vi "Работа с CVS( exel) файлом knob вариант 3.vi"() -> ()   [LabVIEW 2021]
uses:
  CSVtxtcluster.ctl
panel:
  out "record(s)":T1[](array[typedef]) {"Knob" scale=0.0..10.0}
  in  "datalog path (use dialog)":path
  in  "Cluster":T1 {"Knob" scale=0.0..10.0}
  in  "Knob":dbl(knob) scale=0.0..10.0
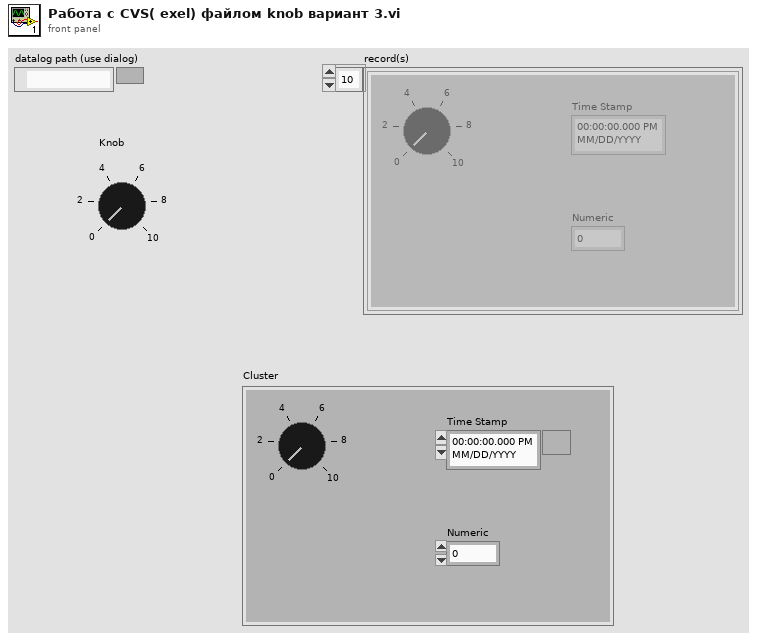
[diagram p1: front panel]
types:
  T1 = typedef "CSVtxtcluster.ctl" = cluster{"Knob":dbl, "Time Stamp":timestamp, "Numeric":dbl}
  T2 = enum16{"open", "replace", "create", "open or create", "replace or create", "replace or create with confirmation"}
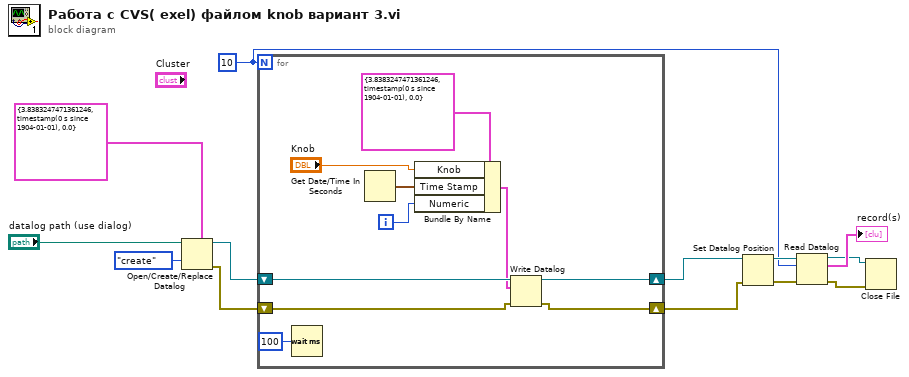
[diagram p0: block diagram]
diagram:
  w3 = 10
  n1 = Open/Create/Replace Datalog(5:T1 {"Knob"=3.8383247471361246, "Time Stamp"=timestamp(0 s since 1904-01-01), "Numeric"=0.0} ("Cluster"), 10:T2."create" ("operation (0:open)"), 11:"datalog path (use dialog)") -> (0:w13:errorcluster, 3:w12:refnum<k1>)  [unwired: 3 in, 1 out]
  n2 = for {
    N: w3 -> [_]
    shift-right: [w22] -> w4
    shift-left: w13 -> [w21]
    shift-right: [w16] -> w6
    shift-left: w12 -> [w15]
    i -> [w19]
    n3 = Wait (ms)(milliseconds to wait=u32 100) -> ()  [unwired: 1 out]
    n4 = Get Date/Time In Seconds() -> (seconds since 1Jan1904=w18:timestamp)
    n5 = Bundle By Name(cluster=T1 {"Knob"=3.8383247471361246, "Time Stamp"=timestamp(0 s since 1904-01-01), "Numeric"=0.0} ("Cluster"), "Knob"="Knob", "Time Stamp"=w18, "Numeric"=w19) -> (w14:T1)
    n6 = Write Datalog(4:w21, 6:w14, 7:w15) -> (0:w22:errorcluster, 3:w16:refnum<k1>)
  }
  n7 = Set Datalog Position(4:w4, 7:w6) -> (0:w7:errorcluster, 3:w5:refnum<k1>)  [unwired: 2 in]
  n8 = Read Datalog(4:w7, 6:w3, 7:w5) -> (0:w2:errorcluster, 2:→"record(s)":T1[], 3:w1:refnum<k1>)
  n9 = Close File(refnum=w1, error in=w2) -> ()  [unwired: 2 out]
